vi "EX 9-5 LEDPWM XBOX.vi"() -> ()   [LabVIEW 2011]
uses:
  <vilib>/LabVIEW Interface for Arduino/Type Defs/Board Type.ctl
  <vilib>/LabVIEW Interface for Arduino/Type Defs/Connection Type.ctl
  <vilib>/LabVIEW Interface for Arduino/Type Defs/Pin Mode.ctl
  <vilib>/Utility/inputDevices.llb/closeJoystick.vi
  <vilib>/Utility/inputDevices.llb/joystickAcquire.vi
  <vilib>/LabVIEW Interface for Arduino/LabVIEW Interface for Arduino.lvlib
panel:
  out "axis info":T1
  out "PWM":i32
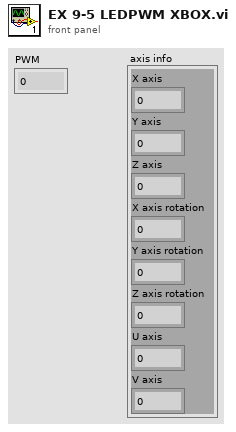
[diagram p1: front panel]
types:
  T1 = cluster{"X axis":i32, "Y axis":i32, "Z axis":i32, "X axis rotation":i32, "Y axis rotation":i32, "Z axis rotation":i32, "U axis":i32, "V axis":i32}
  T2 = typedef "LabVIEW Interface for Arduino.lvlib/Pin Mode.ctl" = enum8{"Input", "Output"}
  T3 = typedef "LabVIEW Interface for Arduino.lvlib/Connection Type.ctl" = enum8{"USB / Serial", "XBEE", "BlueSmirf (Bluetooth)"}
  T4 = typedef "LabVIEW Interface for Arduino.lvlib/Board Type.ctl" = enum16{"Uno", "Dimuelanove w/Atmega 328", "Mega 2560"}
  T5 = typedef "LabVIEW Interface for Arduino.lvlib/Arduino Resource.ctl" = cluster{"VISA resource":refnum<visa-resource-name>, "Board Type":T4, "Connection Type":enum8{"USB / Serial"}, "Bytes Per Packet (15)":u8}
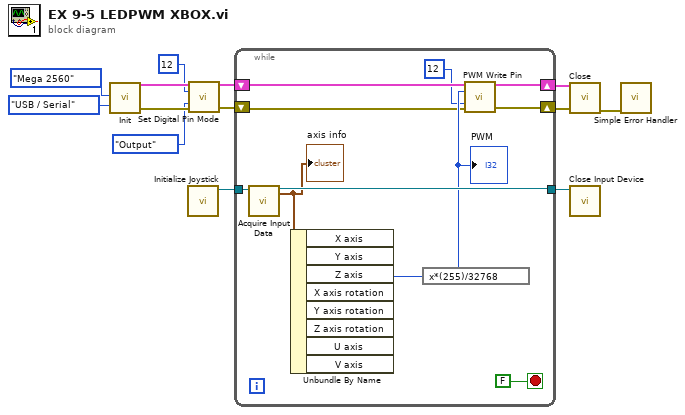
[diagram p0: block diagram]
diagram:
  n1 = call <vilib>:"Init.vi"("Board Type (Uno)"=Board_Type."Mega 2560", "Connection Type (USB/Serial)"=Connection_Type."USB / Serial") -> ("Arduino Resource"=w6:T5, "error out"=w4:errorcluster)  [unwired: 16 in]
  n2 = call <vilib>:"Initialize Joystick.vi"() -> ("device ID"=w8:refnum<k1>)  [unwired: 10 in, 1 out]
  n3 = call <vilib>:"Set Digital Pin Mode.vi"("Arduino Resource"=w6, "Digital I/O Pin"=u8 12, "Pin Mode (Input)"=Pin_Mode."Output", "error in"=w4) -> ("Arduino Resource"=w5:T5, "error out"=w3:errorcluster)  [unwired: 10 in]
  n4 = while {
    shift-right: [w23] -> w13
    shift-left: w5 -> [w16]
    shift-right: [w22] -> w12
    shift-left: w3 -> [w15]
    tunnel: w8 -> [w21]
    tunnel: [w20] -> w7
    stop <- FALSE stop-if-true
    n5 = call-poly <vilib>:"Acquire Input Data.vi"("device ID"=w21) -> ("device ID"=w20:refnum<k1>, "axis info"=w19:T1)  [unwired: 14 in, 3 out]
    "axis info" <- w19
    n6 = Unbundle By Name(w19) -> ("Z axis"=w17:i32)  [unwired: 7 out]
    n7 = expression code="x*(255)/32768"(w17) -> (w18:i32)
    "PWM" <- w18
    n8 = call <vilib>:"PWM Write Pin.vi"("Arduino Resource"=w16, "Duty Cycle (0 - 255)"=w18, "PWM Pin (3)"=u8 12 ("Digital I/O Pin"), "error in"=w15) -> ("Arduino Resource"=w23:T5, "error out"=w22:errorcluster)  [unwired: 10 in]
  }
  n9 = call <vilib>:"Close.vi"("Arduino Resource"=w13, "error in"=w12) -> ("error out"=w11:errorcluster)  [unwired: 13 in]
  n10 = call-poly <vilib>:"Close Input Device.vi"("device ID"=w7) -> ()  [unwired: 9 in, 1 out]
  n11 = call <vilib>:"Simple Error Handler.vi"("error in (no error)"=w11) -> ()  [unwired: 4 in, 5 out]
